vi "Yokogawa - write file.vi"(8 "error in (no error)":errorcluster, 9 "Logging Path":path, 10 "Electrical Data":T1, 11 "Metadata":string[][](array[string])) -> (0 "error out":errorcluster, 3 "file path out":path)   [LabVIEW 2014, in "Yokogawa.lvlib" / "YKPZ400 Logging.lvlib"]
doc: "Save data logged from analyzer to *.tdms file"
uses:
  YKPZ400 Logging.lvlib
  controls/electrical2.ctl
  Acquisition/YKPZ400 Acquisition.lvlib
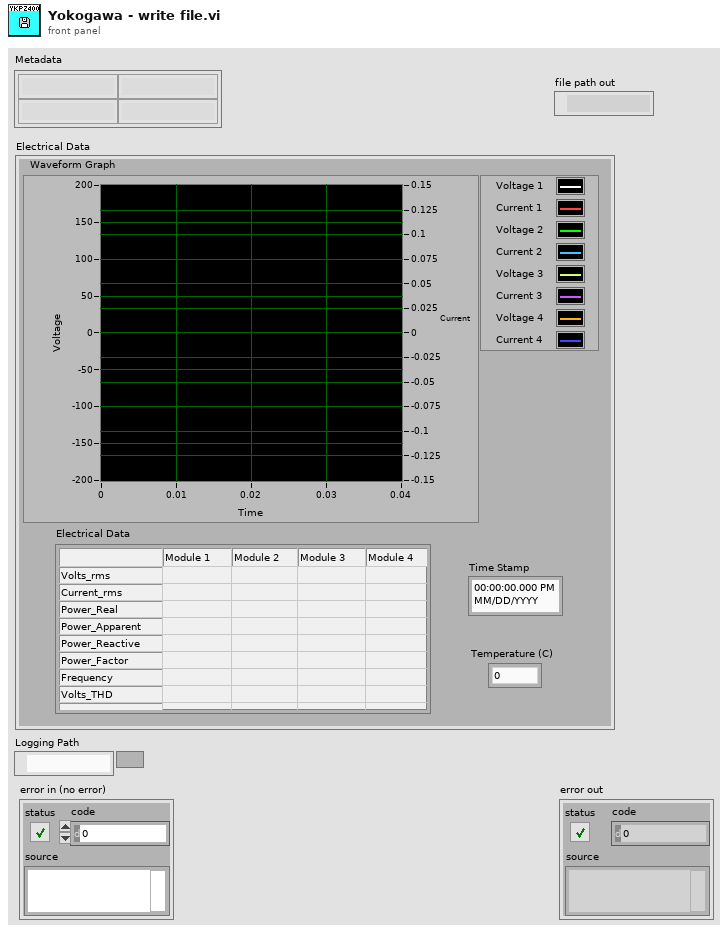
[diagram p1: front panel]
types:
  T1 = typedef "Yokogawa.lvlib/YKPZ400 Acquisition.lvlib/electrical2.ctl" = cluster{"Time Stamp":timestamp, "Temperature (C)":dbl, "Electrical Data":string[][], "Waveform Graph":waveform(dbl)[]}
  T2 = enum16{"open", "open or create", "create or replace", "create", "open (read-only)"}
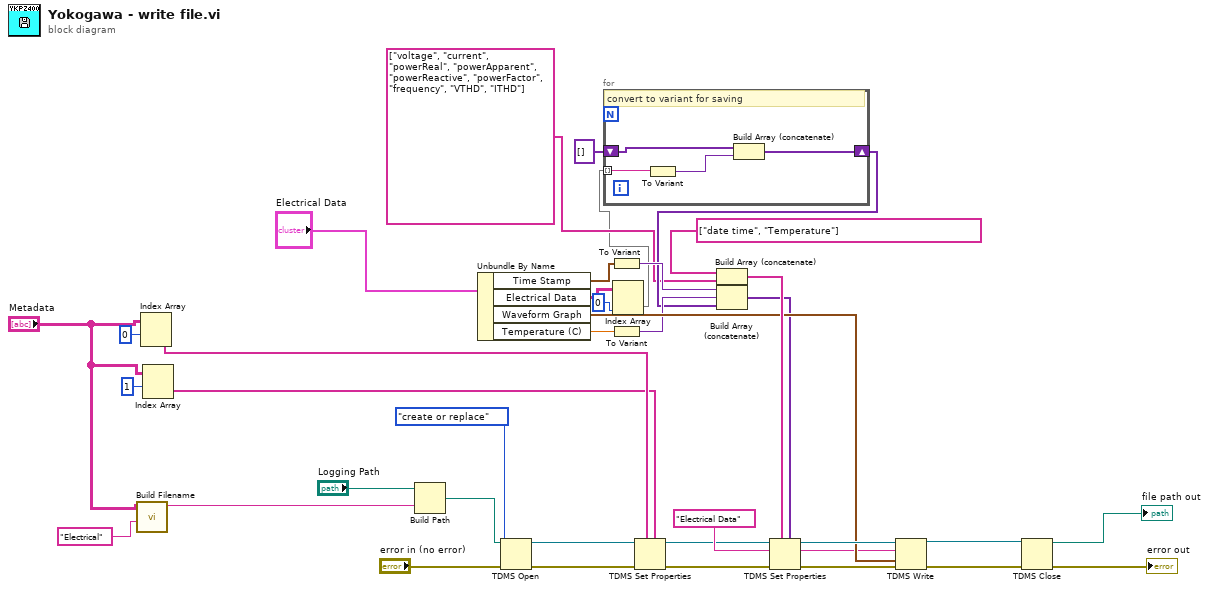
[diagram p0: block diagram]
diagram:
  n1 = call "Build Filename.vi"("Measurment Type"="Electrical", "Metadata In"="Metadata") -> ("String"=w1:string)  [unwired: 9 in]
  n2 = Index Array(array="Metadata", index (row)=0) -> (element=w22:string[])  [unwired: 1 in]
  n3 = Index Array(array="Metadata", index (row)=1) -> (element=w21:string[])  [unwired: 1 in]
  n4 = Build Path(base path="Logging Path", name or relative path=w1) -> (appended path=w2:path)
  n5 = Unbundle By Name("Electrical Data") -> ("Time Stamp"=w13:timestamp, "Electrical Data"=w9:string[][], "Waveform Graph"=w32:waveform(dbl)[], "Temperature (C)"=w20:dbl)
  n6 = TDMS Open(8:"error in (no error)", 10:T2."create or replace" ("operation (0:open)"), 11:w2) -> (0:w25:errorcluster, 3:w26:refnum<k34>)  [unwired: 4 in]
  n7 = To Variant(anything=w13) -> (Variant=w18:variant)
  n8 = To Variant(anything=w20) -> (Variant=w17:variant)
  n9 = Index Array(array=w9, index (col)=0 ("index (row)")) -> (element=w10:string[])  [unwired: 1 in]
  n10 = for {
    tunnel: w10 -> [w42] mode=indexing
    shift-right: [w41] -> w16
    shift-left: variant[] [] -> [w39]
    # "convert to variant for saving"
    n11 = To Variant(anything=w42) -> (Variant=w40:variant)
    n12 = Build Array (concatenate)(w39, w40) -> (w41:variant[])
  }
  n13 = TDMS Set Properties(5:w21, 7:w22, 8:w25, 11:w26) -> (0:w23:errorcluster, 3:w24:refnum<k34>)  [unwired: 2 in, 2 out]
  n14 = Build Array (concatenate)(string[] ["date time", "Temperature"] ("element"), string[] ["voltage", "current", "powerReal", "powerApparent", "powerReactive", "powerFactor", "frequency", "VTHD", "ITHD"]) -> (w33:string[])
  n15 = Build Array (concatenate)(w18, w17, w16) -> (w19:variant[])
  n16 = TDMS Set Properties(5:w19, 7:w33, 8:w23, 10:"Electrical Data" ("group name"), 11:w24) -> (0:w37:errorcluster, 2:w27:string, 3:w38:refnum<k34>)  [unwired: 1 in, 1 out]
  n17 = TDMS Write(0:w38, 5:w27, 9:w32, 11:w37) -> (4:w36:refnum<k34>, 15:w35:errorcluster)  [unwired: 2 in, 2 out]
  n18 = TDMS Close(8:w35, 11:w36) -> (0:→"error out":errorcluster, 3:→"file path out":path)
